vi "Test_API_LogItemDataSource_EventSourceMatch.vi"(8 "error in (no error)":errorcluster, 11 "TestCase in":refnum<class "TestComposedLog.lvclass">) -> (0 "error out":errorcluster, 3 "TestCase out":refnum<class "TestComposedLog.lvclass">)   [LabVIEW 2017, in "TestComposedLog.lvclass"]
uses:
  TestComposedLog.lvclass
  Source/Composed Log/Types/Log Level.ctl
  Source/Composed Log/LoggerReference/LoggerReference.lvclass/LoggerReference.ctl
  Source/LVQueue Sink/LVQueue Sink.lvclass/LVQueue Sink.ctl
  26ac907e-b197-4f92-b50b-edca335a3ee8.vi
  26ac907e-b197-4f92-b50b-edca335a3ee8.vi/98f69271-1de1-4081-8ac1-8b840b0807ac.vi
  Source/Composed Log/LoggerReference/Return Aggregate Queues.vi
  Source/Composed Log/LoggerReference/Add Aggregate Log.vi
  26ac907e-b197-4f92-b50b-edca335a3ee8.vi/98f69271-1de1-4081-8ac1-8b840b0807ac.vi/bbd2f978-e444-4445-9202-4eeb40a61ae4.vi
  Source/Composed Log/LoggerReference/Log.vi
  Source/Composed Log/LoggerReference/Send Add Sink.vi
  Source/Composed Log/LoggerReference/Remove Stale Logs.vi
  Source/LVQueue Sink/LVQueue Sink.lvclass
  C:/CS/Internal/LabVIEW/Logger/Source/Composed Log/Log Sink/Log Sink.lvclass
  Source/Composed Log/Application Logger/Launch Worker Loop.vi
  Source/Composed Log/LoggerReference/Initialize Logger Instance.vi
  Source/Composed Log/Singleton Event Log/Logger Queue FGV.vi
  Source/Composed Log/IErrorFormat/IErrorFormat.lvclass
  Source/Composed Log/LoggerReference/LoggerReference.lvclass
  Source/Composed Log/Log Sink/Log Sink.lvclass
  <vilib>/addons/_JKI Toolkits/VI Tester/TestCase.llb/TestCase.lvclass
  Source/Composed Log/Singleton Event Log/Singleton Event Log.lvlib
  Source/Composed Log/Composed Log.lvlib
  C:/Program Files (x86)/National Instruments/LabVIEW 2017/vi.lib/addons/_JKI Toolkits/VI Tester/TestCase.llb/TestCase.lvclass
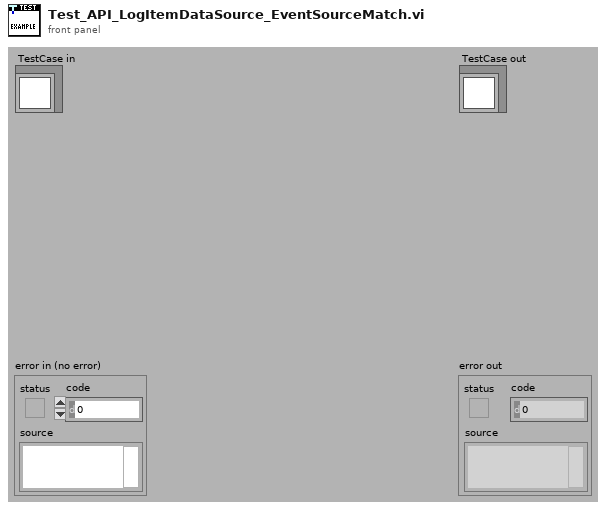
[diagram p1: front panel]
types:
  T1 = typedef "Composed Log.lvlib/Log Level.ctl" = enum16{"Debug", "Info", "Warning", "Error", "Critical"}
  T2 = typedef "Composed Log.lvlib/Log Packet.ctl" = cluster{"Data To Log":string, "Source":string, "Event Level":T1, "Event Time":timestamp}
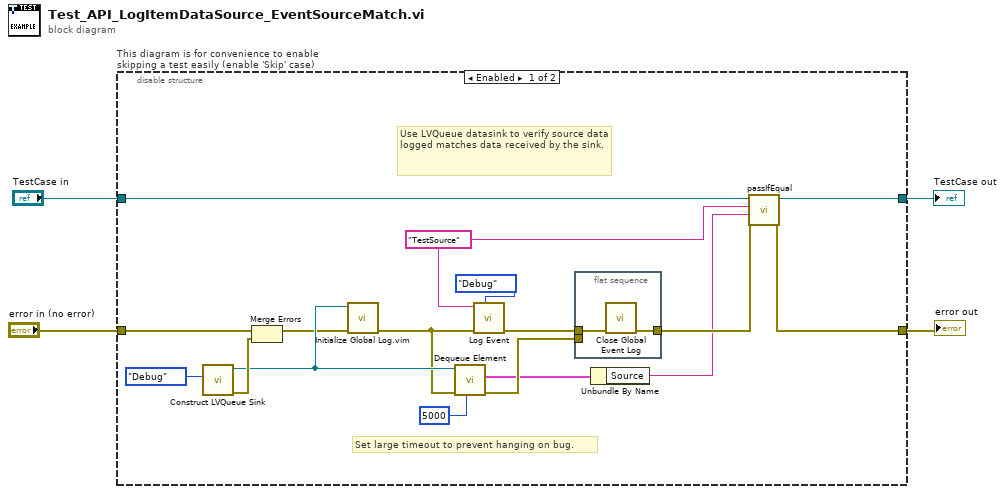
[diagram p0: block diagram]
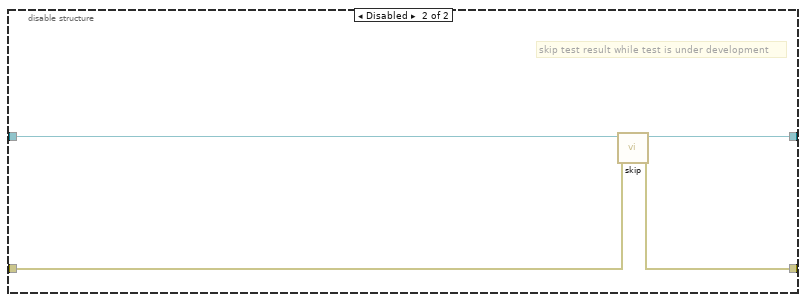
[diagram p2: hidden frame]
diagram:
  n1 = disable-structure "This diagram is for convenience to enable skipping a test easily (enable 'Skip' case)" shown="Enabled" {
    disable-tunnel: "TestCase in" -> [w19 w27]
    disable-tunnel: [w20 w25] -> w1
    disable-tunnel: [w18 w26] -> w3
    disable-tunnel: "error in (no error)" -> [w21 w24]
    frame Enabled {
      w5 = "TestSource" ("Data To Log")
      # "Set large timeout to prevent hanging on bug."
      # "Use LVQueue datasink to verify source data logged matches data received by the sink."
      n2 = call "Construct LVQueue Sink.vi"("LogLevel"=Log_Level."Debug") -> ("error out"=w11:errorcluster, "LVQueue Sink out"=w10:refnum<class "LVQueue Sink.lvclass">)  [unwired: 9 in]
      n3 = Merge Errors(w21, w11) -> (w9:errorcluster)
      n4 = call "Initialize Global Log.vim"("error in (no error)"=w9, "Log Sink(s)"=w10) -> ("error out"=w8:errorcluster)  [unwired: 8 in, 1 out]
      n5 = call "Dequeue Element.vi"("timeout in ms (-1)"=5000, "error in (no error)"=w8, "LVQueue Sink in"=w10) -> ("error out"=w15:errorcluster, "Log Packet"=w13:T2)  [unwired: 5 in, 2 out]
      n6 = call "Log Event.vi"("Event Level"=Log_Level."Debug", "error in (no error)"=w8, "SourceID"=w5) -> ("error out"=w6:errorcluster)  [unwired: 8 in]
      n7 = flat-sequence {
        tunnel: [w23] -> w14
        tunnel: w6 -> [w22]
        tunnel: w15 -> [_]
        frame #0 {
          n8 = call "Close Global Event Log.vi"("error in (no error)"=w22) -> ("error out"=w23:errorcluster)  [unwired: 10 in]
        }
      }
      n9 = Unbundle By Name(w13) -> ("Source"=w12:string)
      n10 = call-dynamic "passIfEqual.vi"("error in (no error)"=w14, "y"=w12, "x"=w5, "TestCase in"=w19) -> ("error out"=w18:errorcluster, "TestCase out"=w20:refnum<class "TestComposedLog.lvclass">)  [unwired: 6 in]
    }
    frame Disabled {
      # "skip test result while test is under development"
      n11 = call <vilib>:"skip.vi"("error in (no error)"=w24, "TestCase in"=w27) -> ("error out"=w26:errorcluster, "TestCase out"=w25:refnum<class "TestComposedLog.lvclass">)  [unwired: 8 in]
    }
  }
  "error out" <- w3
  "TestCase out" <- w1
